vi "Read.vi"(8 "error in (no error)":errorcluster, 10 "Byte Count":u32, 11 "VISA resource name":refnum<visa-resource-name>) -> (0 "error out":errorcluster, 1 "Return Count":u32, 2 "Read Buffer":string, 3 "VISA resource name out":refnum<visa-resource-name>)   [LabVIEW 2023, in "TCxxxx.lvlib"]
uses:
  TCxxxx.lvlib
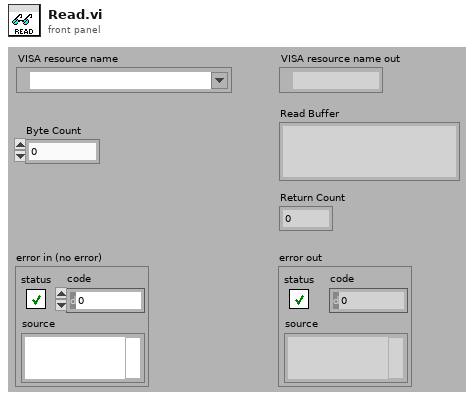
[diagram p1: front panel]
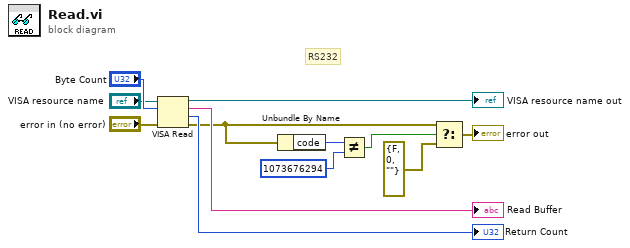
[diagram p0: block diagram]
diagram:
  # "RS232"
  n1 = VISA Read(VISA resource name="VISA resource name", byte count="Byte Count", error in (no error)="error in (no error)") -> (VISA resource name out=→"VISA resource name out":refnum<visa-resource-name>, read buffer=→"Read Buffer":string, return count=→"Return Count":u32, error out=w3:errorcluster)
  n2 = Unbundle By Name(w3) -> ("code"=w7:i32)
  n3 = Not Equal?(x=w7, y=1073676294) -> (x != y?=w4:bool)
  n4 = Select(t=w3, s=w4, f=errorcluster {"status"=FALSE, "code"=0, "source"=""} ("error out")) -> (s? t:f=→"error out":errorcluster)
